vi "picoquant_fifo_loop.vi"(8 "error in (no error)":errorcluster, 11 "picoquant_generic in":refnum<class "picoquant_generic.lvclass">) -> (0 "error out":errorcluster, 3 "picoquant_generic out":refnum<class "picoquant_generic.lvclass">)   [LabVIEW 2015, in "picoquant_generic.lvclass"]
uses:
  picoquant_generic.lvclass
  loop_notifier_tdef.ctl
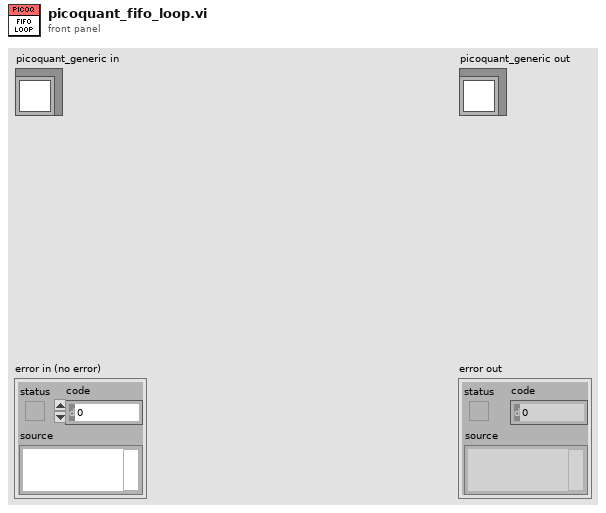
[diagram p1: front panel]
types:
  T1 = typedef "loop_notifier_tdef.ctl" = enum16{"exit"}
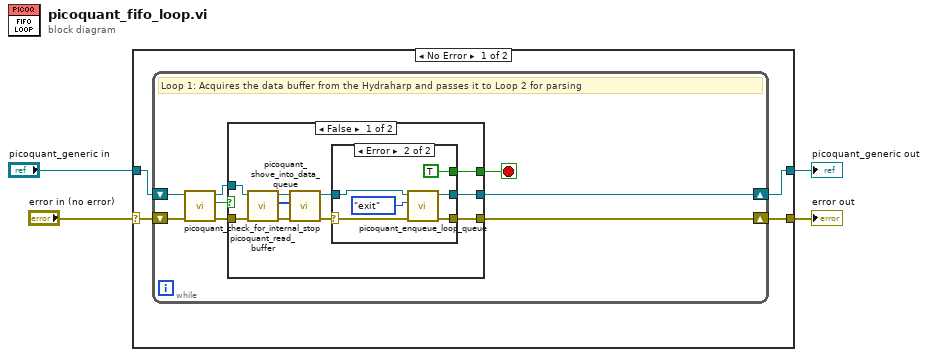
[diagram p0: block diagram]
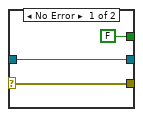
[diagram p2: hidden frame]
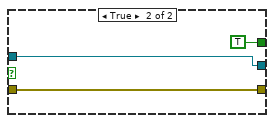
[diagram p3: hidden frame]
diagram:
  n1 = case shown="No Error" "error in (no error)" {
    selector: "error in (no error)" -> [w7 w40]
    tunnel: [w6 w40] -> w3
    tunnel: [w5 w39] -> w1
    tunnel: "picoquant_generic in" -> [w8 w39]
    frame No Error {
      n2 = while {
        shift-right: [w11] -> w5
        shift-left: w8 -> [w15]
        shift-right: [w12] -> w6
        shift-left: w7 -> [w16]
        stop <- w9 stop-if-true
        # "Loop 1: Acquires the data buffer from the Hydraharp and passes it to Loop 2 for parsing"
        n3 = call "picoquant_check_for_internal_stop.vi"("error in (no error)"=w16, "picoquant_generic in"=w15) -> ("error out"=w13:errorcluster, "exit?"=w10:bool, "picoquant_generic out"=w14:refnum<class "picoquant_generic.lvclass">)  [unwired: 7 in]
        n4 = case shown="False" w10 {
          tunnel: w14 -> [w26 w37]
          tunnel: w13 -> [w25 w36]
          tunnel: [w20 w36] -> w12
          tunnel: [w17 w37] -> w11
          tunnel: [w19 TRUE] -> w9
          frame False {
            n5 = call-dynamic "picoquant_read_buffer.vi"("error in (no error)"=w25, "picoquant_generic in"=w26) -> ("error out"=w24:errorcluster, "new_data"=w22:u32[], "picoquant_generic out"=w23:refnum<class "picoquant_generic.lvclass">)  [unwired: 7 in]
            n6 = call "picoquant_shove_into_data_queue.vi"("error in (no error)"=w24, "new_data"=w22, "picoquant_generic in"=w23) -> ("error out"=w21:errorcluster, "picoquant_generic out"=w18:refnum<class "picoquant_generic.lvclass">)  [unwired: 7 in]
            n7 = case shown="Error" w21 {
              selector: w21 -> [w29 w33]
              tunnel: [w29 w32] -> w20
              tunnel: [FALSE TRUE] -> w19
              tunnel: w18 -> [w27 w35]
              tunnel: [w27 w34] -> w17
              frame No Error {
              }
              frame Error {
                n8 = call "picoquant_enqueue_loop_queue.vi"("error in (no error)"=w33, "loop_notifier"=loop_notifier_tdef."exit" ("element"), "picoquant_generic in"=w35) -> ("error out"=w32:errorcluster, "picoquant_generic out"=w34:refnum<class "picoquant_generic.lvclass">)  [unwired: 7 in]
              }
            }
          }
          frame True {
          }
        }
      }
    }
    frame Error {
    }
  }
  "error out" <- w3
  "picoquant_generic out" <- w1
